vi "stimulate.vi"(0 "force base":bool, 2 "vars in":T1={"wait count t"=0, "wait min"=0, "wait max"=0, "stim count t"=0, "stim count n"=0, "d stim"=0, "d timeout"=0, "timeout win"=0, "base temp"=0.0, "stim amps"=[], "n hit"=0, "n catch"=0, "active"=TRUE, "catch"=TRUE, "stimulus"=TRUE, "reward given"=TRUE, "pairing"=TRUE, "lick"=FALSE, "next reward"=FALSE, "clean tubes"=FALSE, "next temp"=0.0}) -> (7 "vars out":T1={"wait count t"=0, "wait min"=0, "wait max"=0, "stim count t"=0, "stim count n"=0, "d stim"=0, "d timeout"=0, "timeout win"=0, "base temp"=0.0, "stim amps"=[], "n hit"=0, "n catch"=0, "active"=TRUE, "catch"=TRUE, "stimulus"=TRUE, "reward given"=TRUE, "pairing"=TRUE, "lick"=FALSE, "next reward"=FALSE, "clean tubes"=FALSE, "next temp"=0.0})   [LabVIEW 2015]
uses:
  Type Definitions/vars.ctl
panel:
  # "(see Block Diagram)"
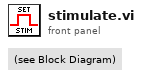
[diagram p1: front panel]
types:
  T1 = typedef "vars.ctl" = cluster{"wait count t":u16, "wait min":u16, "wait max":u16, "stim count t":u16, "stim count n":u16, "d stim":u16, "d timeout":u16, "timeout win":u16, "base temp":sgl, "stim amps":i32[], "n hit":u16, "n catch":u16, "active":bool, "catch":bool, "stimulus":bool, "reward given":bool, "pairing":bool, "lick":bool, "next reward":bool, "clean tubes":bool, "next temp":sgl}
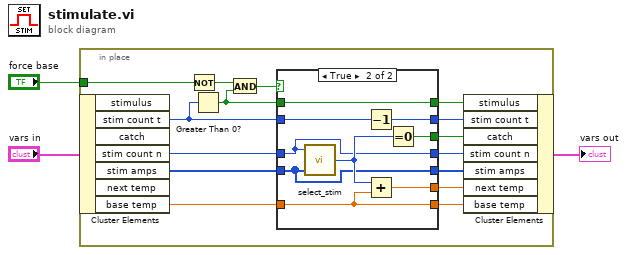
[diagram p0: block diagram]
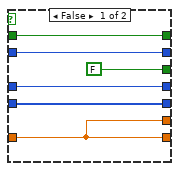
[diagram p2: hidden frame]
diagram:
  n1 = in-place {
    in-place-border: "force base" -> [w5]
    n2 = in-place-cluster #1("vars in") -> ("stim count t"=w16:u16, "stim count n"=w14:u16, "stim amps"=w13:i32[], "base temp"=w12:sgl)  [unwired: 3 out]
    n3 = Not(x=w5) -> (.not. x?=w17:bool)
    n4 = Greater Than 0?(x=w16) -> (x > 0?=w4:bool)
    n5 = And(x=w17, y=w4) -> (x .and. y?=w18:bool)
    n6 = case shown="True" w18 {
      tunnel: w16 -> [w24 w33]
      tunnel: [w24 w32] -> w15
      tunnel: w12 -> [w22 w28]
      tunnel: [w22 w31] -> w11
      tunnel: [w19 w25] -> w6
      tunnel: [FALSE w30] -> w9
      tunnel: w14 -> [w20 w26]
      tunnel: w13 -> [w21 w27]
      tunnel: [w22 w28] -> w10
      tunnel: [w21 w27] -> w8
      tunnel: [w20 w26] -> w7
      tunnel: w4 -> [w19 w25]
      frame False {
      }
      frame True {
        n7 = call "select_stim.vi"("stim count"=w27, "stim array"=w26) -> ("stim"=w29:i32)  [unwired: 1 in]
        n8 = Decrement(x=w33) -> (x-1=w32:u16)
        n9 = Add(x=w29, y=w28) -> (x+y=w31:sgl)
        n10 = Equal To 0?(x=w29) -> (x = 0?=w30:bool)
      }
    }
    n11 = in-place-cluster #1("stimulus"=w6, "stim count t"=w15, "catch"=w9, "stim count n"=w7, "stim amps"=w8, "next temp"=w11, "base temp"=w10) -> (→"vars out":T1)
  }
